vi "testTwoServersReportInternalError.vi"(8 "error in":errorcluster) -> (0 "error out":errorcluster)   [LabVIEW 2018]
uses:
  <vilib>/addons/_JKI Toolkits/Caraya/classes/Assert/Assert Not Equal Value_Variant.vi
  src/TcpServer/TcpServer.lvclass
  <vilib>/addons/_JKI Toolkits/Caraya/classes/Test/Test.lvclass
  <vilib>/addons/_JKI Toolkits/Caraya/classes/Assert/Assert.lvclass
panel:
  in  "logNow":bool
  out "Run Server B error":errorcluster
  out "Run Server A error":errorcluster
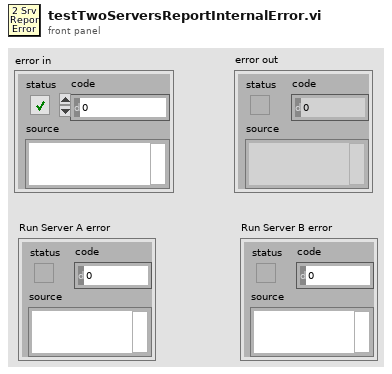
[diagram p1: front panel]
types:
  T1 = cluster{"CmdRead":refnum<user-event>, "EvtRead":refnum<user-event>, "GenRead":refnum<user-event>}
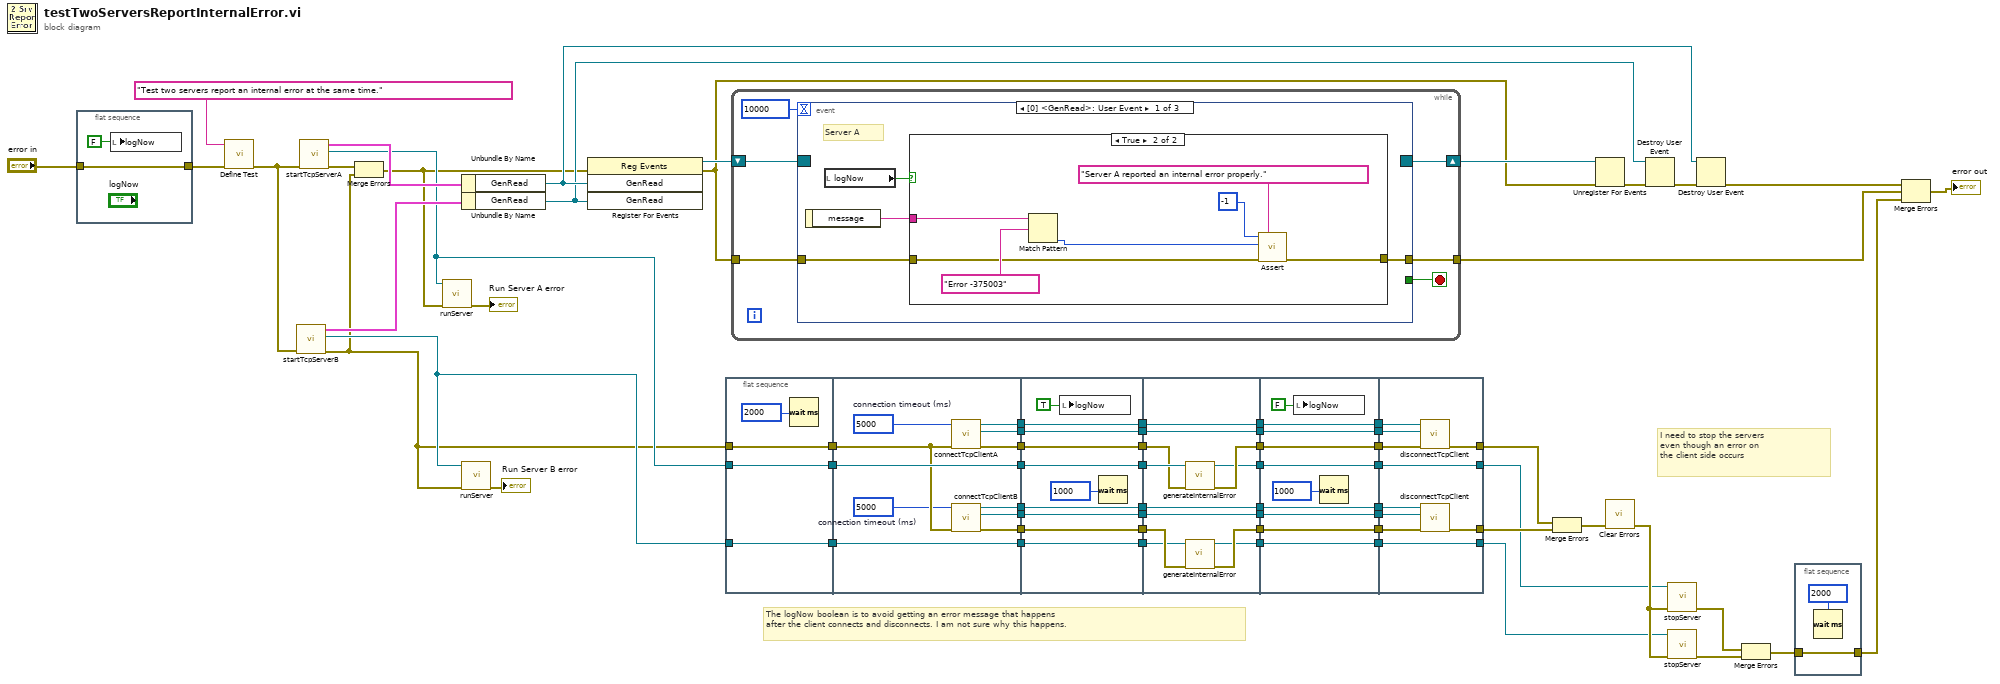
[diagram p0: block diagram]
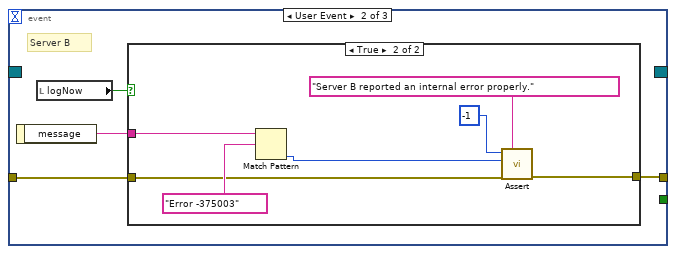
[diagram p3: hidden frame]
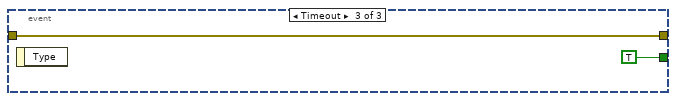
[diagram p5: hidden frame]
diagram:
  # "The logNow boolean is to avoid getting an error message that happens\nafter the client connects and disconnects. I am not sure why this happens."
  # "Event Structure for TCP server B"
  # "Event Structure for TCP server A"
  # "I need to stop the servers \neven though an error on \nthe client side occurs"
  n1 = flat-sequence {
    tunnel: [w69] -> w5
    tunnel: "error in" -> [w69]
    frame #0 {
      n2 = local write "logNow"(FALSE ("logNow")) -> ()
    }
  }
  n3 = call <vilib>:"Define Test.vi"("error in (no error)"=w5, "Label (VI Title)"="Test two servers report an internal error at the same time.") -> ("error out"=w63:errorcluster)  [unwired: 9 in]
  n4 = call "startTcpServerB.vi"("error in (no error)"=w63) -> ("error out"=w1:errorcluster, "TcpServer out"=w48:refnum<class "TcpServer.lvclass">, "UserEvents"=w61:T1)  [unwired: 8 in]
  n5 = call "startTcpServerA.vi"("error in (no error)"=w63) -> ("error out"=w50:errorcluster, "TcpServer out"=w15:refnum<class "TcpServer.lvclass">, "UserEvents"=w62:T1)  [unwired: 8 in]
  n6 = Merge Errors(w50, w1) -> (w2:errorcluster)
  n7 = call "runServer.vi"("error in (no error)"=w2, "TcpServer in"=w15) -> ("error out (no error)"=→"Run Server A error":errorcluster)  [unwired: 8 in, 1 out]
  n8 = Unbundle By Name(w62) -> ("GenRead"=w7:refnum<user-event>)
  n9 = Unbundle By Name(w61) -> ("GenRead"=w6:refnum<user-event>)
  n10 = call "runServer.vi"("error in (no error)"=w1, "TcpServer in"=w48) -> ("error out (no error)"=→"Run Server B error":errorcluster)  [unwired: 8 in, 1 out]
  n11 = register-events(error in=w2, w7, w6) -> (reference out=w60:refnum<event-registration>, error out=w11:errorcluster)  [unwired: 1 in]
  n12 = flat-sequence {
    tunnel: [w73] -> w59
    tunnel: [w72] -> w49
    tunnel: [w71] -> w47
    tunnel: w1 -> [w73]
    tunnel: w15 -> [w72]
    tunnel: w48 -> [w71]
    tunnel: [w85] -> w45
    tunnel: [w84] -> w43
    tunnel: [w83] -> w41
    tunnel: [w82] -> w39
    tunnel: [w81] -> w37
    tunnel: [w80] -> w35
    tunnel: w59 -> [w78]
    tunnel: w49 -> [w79]
    tunnel: [w79] -> w33
    tunnel: w47 -> [w77]
    tunnel: [w77] -> w31
    tunnel: w45 -> [w95]
    tunnel: [w95] -> w44
    tunnel: w43 -> [w94]
    tunnel: [w94] -> w42
    tunnel: w41 -> [w93]
    tunnel: [w93] -> w40
    tunnel: w39 -> [w92]
    tunnel: [w92] -> w38
    tunnel: w37 -> [w91]
    tunnel: [w91] -> w36
    tunnel: w35 -> [w90]
    tunnel: [w90] -> w34
    tunnel: w33 -> [w89]
    tunnel: [w89] -> w32
    tunnel: w31 -> [w88]
    tunnel: [w88] -> w30
    tunnel: [w107] -> w29
    tunnel: w44 -> [w107]
    tunnel: [w106] -> w27
    tunnel: w42 -> [w106]
    tunnel: w40 -> [w102]
    tunnel: [w105] -> w25
    tunnel: w38 -> [w105]
    tunnel: [w104] -> w23
    tunnel: w36 -> [w104]
    tunnel: [w99] -> w21
    tunnel: w34 -> [w100]
    tunnel: w32 -> [w103]
    tunnel: [w101] -> w19
    tunnel: w30 -> [w98]
    tunnel: [w97] -> w17
    tunnel: [w96] -> w12
    tunnel: w29 -> [w117]
    tunnel: [w117] -> w28
    tunnel: w27 -> [w116]
    tunnel: [w116] -> w26
    tunnel: w25 -> [w115]
    tunnel: [w115] -> w24
    tunnel: w23 -> [w114]
    tunnel: [w114] -> w22
    tunnel: w21 -> [w113]
    tunnel: [w113] -> w20
    tunnel: w19 -> [w112]
    tunnel: [w112] -> w18
    tunnel: w17 -> [w111]
    tunnel: [w111] -> w16
    tunnel: [w109] -> w13
    tunnel: w12 -> [w109]
    tunnel: w28 -> [w127]
    tunnel: w26 -> [w126]
    tunnel: w24 -> [w124]
    tunnel: w22 -> [w123]
    tunnel: w20 -> [w122]
    tunnel: w18 -> [w125]
    tunnel: w16 -> [w119]
    tunnel: w13 -> [w118]
    tunnel: [w121] -> w57
    tunnel: [w120] -> w56
    tunnel: [w119] -> w46
    tunnel: [w118] -> w14
    frame #0 {
      n13 = Wait (ms)(milliseconds to wait=u32 2000) -> ()  [unwired: 1 out]
    }
    frame #1 {
      w75 = 5000  # connection timeout (ms)
      w76 = 5000  # connection timeout (ms)
      n14 = call "connectTcpClientA.vi"("error in (no error)"=w78, "connection timeout (ms)"=w76) -> ("error out"=w83:errorcluster, "tel connection ID A out"=w84:refnum<k5>, "cmd connection ID A out"=w85:refnum<k5>)  [unwired: 7 in]
      n15 = call "connectTcpClientB.vi"("error in (no error)"=w78, "connection timeout (ms)"=w75) -> ("error out"=w80:errorcluster, "tel connection ID B out"=w81:refnum<k5>, "cmd connection ID B out"=w82:refnum<k5>)  [unwired: 7 in]
    }
    frame #2 {
      n16 = local write "logNow"(TRUE ("logNow")) -> ()
      n17 = Wait (ms)(milliseconds to wait=u32 1000) -> ()  [unwired: 1 out]
    }
    frame #3 {
      n18 = call "generateInternalError.vi"("error in (no error)"=w102, "tcpServer in"=w103) -> ("error out"=w101:errorcluster, "tcpServer out"=w96:refnum<class "TcpServer.lvclass">)  [unwired: 8 in]
      n19 = call "generateInternalError.vi"("error in (no error)"=w100, "tcpServer in"=w98) -> ("error out"=w99:errorcluster, "tcpServer out"=w97:refnum<class "TcpServer.lvclass">)  [unwired: 8 in]
    }
    frame #4 {
      n20 = local write "logNow"(FALSE ("logNow")) -> ()
      n21 = Wait (ms)(milliseconds to wait=u32 1000) -> ()  [unwired: 1 out]
    }
    frame #5 {
      n22 = call "disconnectTcpClient.vi"("error in (no error)"=w125, "tel connection ID in"=w126, "cmd connection ID in"=w127) -> ("error out"=w121:errorcluster)  [unwired: 8 in]
      n23 = call "disconnectTcpClient.vi"("error in (no error)"=w122, "tel connection ID in"=w123, "cmd connection ID in"=w124) -> ("error out"=w120:errorcluster)  [unwired: 8 in]
    }
  }
  n24 = while {
    shift-right: [w132] -> w58
    shift-left: w60 -> [w133]
    tunnel: w11 -> [w129]
    tunnel: [w128] -> w10
    stop <- w130 stop-if-true
    n25 = event shown="[0] <GenRead>: User Event" {
      selector: w133 -> [_ _ _]
      dyn-events: [_ _ _] -> w132
      timeout: 10000 -> [_ _ _]
      tunnel: [_ _ TRUE] -> w130
      tunnel: w129 -> [w136 w148 w158]
      tunnel: [w135 w147 w158] -> w128
      event User Event {
        # "Server A"
        n26 = event-data() -> ("message"=w137:string)  [unwired: 1 in]
        n27 = local read "logNow"() -> (w134:bool)
        n28 = case shown="True" w134 {
          tunnel: w137 -> [_ w144]
          tunnel: w136 -> [w138 w142]
          tunnel: [w138 w140] -> w135
          frame False {
          }
          frame True {
            n29 = Match Pattern(string=w144, regular expression="Error -375003" ("error string")) -> (offset past match=w139:i32)  [unwired: 1 in, 3 out]
            n30 = call-poly <vilib>:"Assert.vi"("Label"="Server A reported an internal error properly.", "error in (no error)"=w142, "Y"=w139, "X"=-1 ("offset past match")) -> ("error out"=w140:errorcluster)  [unwired: 7 in]
          }
        }
      }
      event User Event {
        # "Server B"
        n31 = event-data() -> ("message"=w149:string)  [unwired: 1 in]
        n32 = local read "logNow"() -> (w146:bool)
        n33 = case shown="True" w146 {
          tunnel: w149 -> [_ w156]
          tunnel: w148 -> [w150 w154]
          tunnel: [w150 w152] -> w147
          frame False {
          }
          frame True {
            n34 = Match Pattern(string=w156, regular expression="Error -375003" ("error string")) -> (offset past match=w151:i32)  [unwired: 1 in, 3 out]
            n35 = call-poly <vilib>:"Assert.vi"("Label"="Server B reported an internal error properly.", "error in (no error)"=w154, "Y"=w151, "X"=-1 ("offset past match")) -> ("error out"=w152:errorcluster)  [unwired: 7 in]
          }
        }
      }
      event Timeout {
        n36 = event-data() -> ()  [unwired: 1 in, 1 out]
      }
    }
  }
  n37 = Merge Errors(w57, w56) -> (w55:errorcluster)
  n38 = Unregister For Events(event registration refnum=w58, error in=w11) -> (error out=w53:errorcluster)
  n39 = call <vilib>:"Clear Errors.vi"("error in (no error)"=w55) -> ("error out"=w54:errorcluster)  [unwired: 5 in, 1 out]
  n40 = Destroy User Event(user event=w6, error in=w53) -> (error out=w9:errorcluster)
  n41 = call "stopServer.vi"("error in (no error)"=w54, "tcpServer in"=w14) -> ("error out"=w66:errorcluster)  [unwired: 8 in, 1 out]
  n42 = call "stopServer.vi"("error in (no error)"=w54, "tcpServer in"=w46) -> ("error out"=w65:errorcluster)  [unwired: 8 in, 1 out]
  n43 = Destroy User Event(user event=w7, error in=w9) -> (error out=w8:errorcluster)
  n44 = Merge Errors(w66, w65) -> (w64:errorcluster)
  n45 = flat-sequence {
    tunnel: w64 -> [w160]
    tunnel: [w160] -> w51
    frame #0 {
      n46 = Wait (ms)(milliseconds to wait=u32 2000) -> ()  [unwired: 1 out]
    }
  }
  n47 = Merge Errors(w8, w10, w51) -> (→"error out":errorcluster)
